vi "Handle Error.vi"(8 "error in (no error)":errorcluster, 11 "Actor in":refnum<class "Actor.lvclass">) -> (0 "error out":errorcluster, 2 "stop actor?":bool=TRUE, 3 "Actor out":refnum<class "Actor.lvclass">)   [LabVIEW 2017, in "Actor Framework.lvlib" / "Actor.lvclass"]
doc: "(<B>Filename</B>: Actor Framework.lvlib:Actor.lvclass:Handle Error.vi)\n\nDefines how the actor handles an error that occurred while processing a message. By default, this method does nothing except stop the actor."
uses:
  <vilib>/ActorFramework/Actor/Actor.lvclass
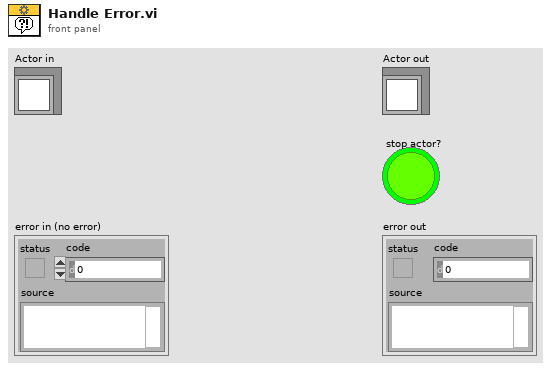
[diagram p1: front panel]
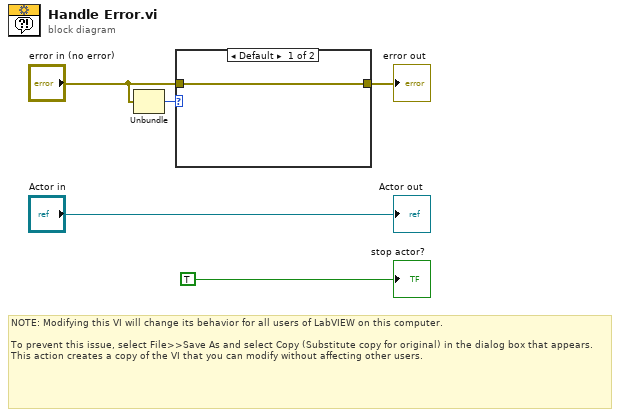
[diagram p0: block diagram]
diagram:
  # "NOTE: Modifying this VI will change its behavior for all users of LabVIEW on this computer.\n\nTo prevent this issue, select File>>Save As and select Copy (Substitute copy for original) in the dialog box that appears. This action creates a copy of the VI that you can modify without affecting other users."
  n1 = Unbundle("error in (no error)") -> ("code"=w5:i32)  [unwired: 2 out]
  n2 = case shown="Default" w5 {
    tunnel: [w6 _] -> w3
    tunnel: "error in (no error)" -> [w6 _]
    frame Default {
    }
    frame 43 {
      # "\"Cancel Error\" means stop, but \"No Error\" to caller."
    }
  }
  "error out" <- w3
  "Actor out" <- "Actor in"
  "stop actor?" <- TRUE
